vi "CreateErrorLog.vi"(8 "error in (no error)":errorcluster {"code" format="Error %.0f"}, 10 "operation (0:open)":T1(ring)=enum."open or create", 11 "RelativePath (ErrorLog.txt)":path=path "ErrorLog.txt") -> (0 "error out":errorcluster {"code" format="Error %.0f"}, 3 "refnum out":refnum<file>)   [LabVIEW 2017]
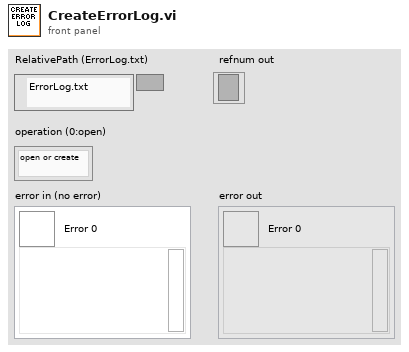
[diagram p1: front panel]
types:
  T1 = enum16{"open", "replace", "create", "open or create", "replace or create", "replace or create with confirmation"}
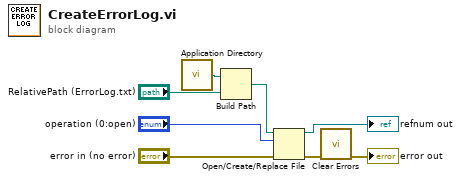
[diagram p0: block diagram]
diagram:
  n1 = call <vilib>:"Application Directory.vi"() -> ("Application Directory"=w7:path)
  n2 = Build Path(base path=w7, name or relative path="RelativePath (ErrorLog.txt)") -> (appended path=w6:path)
  n3 = Open/Create/Replace File(file path (use dialog)=w6, error in="error in (no error)", operation (0:open)="operation (0:open)") -> (refnum out=→"refnum out":refnum<file>, error out=w8:errorcluster)  [unwired: 3 in, 1 out]
  n4 = call <vilib>:"Clear Errors.vi"("error in (no error)"=w8) -> ("error out"=→"error out":errorcluster)  [unwired: 5 in, 1 out]
